vi "Cholesky Factorization Rank-1 Update_Downdate (DBL).vi"(10 "X":dbl[](array[numeric]), 11 "R":T1) -> (0 "error":i32, 3 "Updated R":T1)   [LabVIEW 2020, in "NI_AAL_LinAlg.lvlib"]
uses:
  <vilib>/Analysis/NI_AAL_LinAlg.lvlib
  <vilib>/Analysis/Matrix/Datatypes/RealMatrix.ctl
  <vilib>/Analysis/baseanly.llb/Matrix Type of Inverse Matrix.ctl
  <vilib>/Analysis/7linalg.llb/Real Transpose Matrix.vi
  <vilib>/Analysis/7linalg.llb/Solve Linear Equations (single right hand).vi
  <vilib>/Analysis/baseanly.llb/Unit Vector (DBL).vi
  <vilib>/Analysis/baseanly.llb/Solve Linear Equations By Cholesky.vi
  <vilib>/Analysis/baseanly.llb/Real Matrix to Compact Array.vi
  <vilib>/Analysis/baseanly.llb/Real Compact Tri-Matrix Linear Eqs.vi
  <vilib>/Analysis/7linalg.llb/Solve Linear Eqs (General).vi
  <vilib>/Analysis/7linalg.llb/Solve Linear Eqs (Gen, single right hand).vi
  <vilib>/Analysis/NI_AALBase.lvlib
  <vilib>/Analysis/NI_AALPro.lvlib
  <vilib>/Analysis/Matrix/NI_Matrix.lvlib
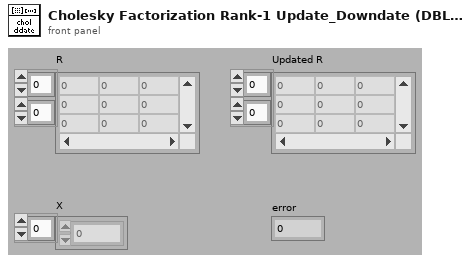
[diagram p1: front panel]
types:
  T1 = typedef "NI_Matrix.lvlib/RealMatrix.ctl" = dbl[][]
  T2 = typedef "NI_AALBase.lvlib/Matrix Type of Inverse Matrix.ctl" = enum32{"General", "Positive Definite", "Lower Triangular", "Upper Triangular"}
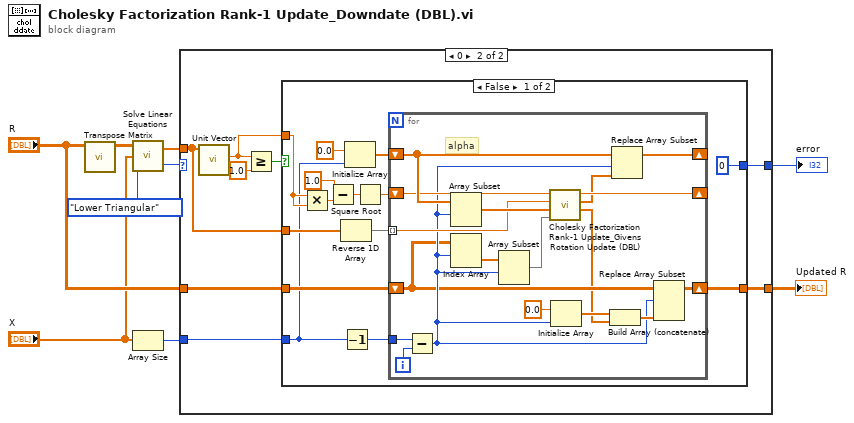
[diagram p0: block diagram]
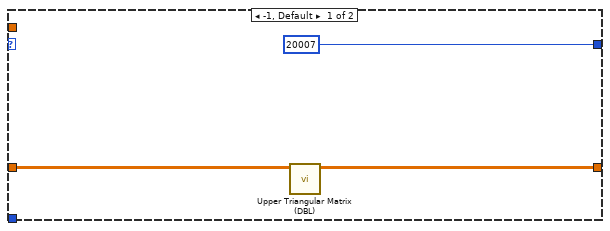
[diagram p2: hidden frame]
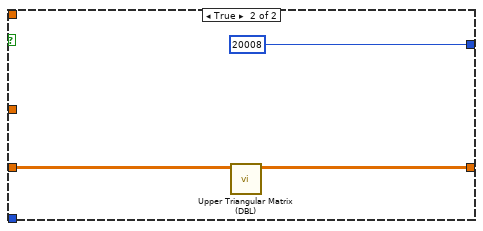
[diagram p3: hidden frame]
diagram:
  n1 = call-poly <vilib>:"Transpose Matrix.vi"("Input Matrix"="R") -> ("Matrix Transpose"=w5:T1)  [unwired: 9 in, 1 out]
  n2 = call-poly <vilib>:"Solve Linear Equations.vi"("matrix type"=Matrix_Type_of_Inverse_Matrix."Lower Triangular", "Known Vector"="X", "Input Matrix"=w5) -> ("error"=w7:i32, "Solution Vector"=w8:dbl[])
  n3 = Array Size(array="X") -> (size(s)=w9:i32)
  n4 = case shown="0" w7 {
    tunnel: w8 -> [_ w14]
    tunnel: "R" -> [w10 w15]
    tunnel: [w11 w18] -> w1
    tunnel: [20007 w17] -> w2
    tunnel: w9 -> [_ w16]
    frame -1, Default {
      n5 = call <vilib>:"Upper Triangular Matrix (DBL).vi"("A"=w10) -> ("U"=w11:T1)  [unwired: 10 in]
    }
    frame 0 {
      n6 = call-poly <vilib>:"Unit Vector.vi"("Input Vector"=w14) -> ("norm"=w13:dbl)  [unwired: 2 in, 8 out]
      n7 = Greater Or Equal?(x=w13, y=1.0) -> (x >= y?=w19:bool)
      n8 = case shown="False" w19 {
        tunnel: w14 -> [w30 _]
        tunnel: w13 -> [w34 _]
        tunnel: w15 -> [w28 w53]
        tunnel: [w22 w54] -> w18
        tunnel: [0 20008] -> w17
        tunnel: w16 -> [w24 _]
        frame False {
          n9 = Multiply(x=w34, y=w34) -> (x*y=w33:dbl)
          n10 = Subtract(x=1.0, y=w33) -> (x-y=w26:dbl)
          n11 = Reverse 1D Array(array=w30) -> (reversed array=w23:dbl[])
          n12 = Decrement(x=w24) -> (x-1=w31:i32)
          n13 = Initialize Array(0.0 ("x+y"), w24) -> (w29:dbl[])
          n14 = Square Root(x=w26) -> (sqrt(x)=w25:dbl)
          n15 = for {
            shift-right: [w38] -> _
            shift-left: w25 -> [w46]
            tunnel: w31 -> [w52]
            tunnel: w23 -> [w43] mode=indexing
            shift-right: [w49] -> _
            shift-left: w29 -> [w50]
            shift-right: [w39] -> w22
            shift-left: w28 -> [w40]
            i -> [w51]
            # "alpha"
            n16 = Subtract(x=w52, y=w51) -> (x-y=w41:i32)
            n17 = Array Subset(array=w50, index=w41) -> (w45:dbl[])  [unwired: 1 in]
            n18 = Index Array(array=w40, index (row)=w41) -> (element=w47:dbl[])  [unwired: 1 in]
            n19 = Array Subset(array=w47, index=w41) -> (w44:dbl[])  [unwired: 1 in]
            n20 = call <vilib>:"Cholesky Factorization Rank-1 Update_Givens Rotation Update (DBL).vi"("Y In"=w44, "X In"=w45, "b"=w43, "a"=w46) -> ("Y Out"=w35:dbl[], "X Out"=w36:dbl[], "v"=w38:dbl)  [unwired: 5 in]
            n21 = Initialize Array(0.0 ("element"), w41) -> (w48:dbl[])
            n22 = Build Array (concatenate)(w48, w35) -> (w42:dbl[])
            n23 = Replace Array Subset(array=w50, new element=w36, index=w41) -> (w49:dbl[])
            n24 = Replace Array Subset(array=w40, new element=w42, index (row)=w41) -> (w39:T1)  [unwired: 1 in]
          }
        }
        frame True {
          n25 = call <vilib>:"Upper Triangular Matrix (DBL).vi"("A"=w53) -> ("U"=w54:T1)  [unwired: 10 in]
        }
      }
    }
  }
  "Updated R" <- w1
  "error" <- w2
